vi "Actor Core.vi"(8 "error in":errorcluster, 11 "Example View in":refnum<class "Example View Actor 2.lvclass">) -> (0 "error out":errorcluster, 3 "Actor out":refnum<class "Actor.lvclass">)   [LabVIEW 2023, in "Example Event Actors.lvlib" / "Example View Actor 2.lvlib" / "Example View Actor 2.lvclass"]
doc: "(<B>Filename</B>: Actor Framework.lvlib:Actor.lvclass:Actor Core.vi)\n\nReceives messages to the actor, reacts to them, and initiates any error handling that may shut the actor down.\n\nDescendant classes may override this VI to append parallel tasks for the actor to complete while it handles messages. Overrides use the Call Parent Method node."
uses:
  Example View Actor 2.lvclass
  C:/Program Files/National Instruments/LabVIEW 2023/vi.lib/ActorFramework/Actor/Actor.lvclass
  C:/Projects/Shared Libraries/Event Actors/View Actor/View Actor.lvclass
  <vilib>/ActorFramework/Actor/Actor.lvclass
  Example View Actor 2.lvclass/Example View Actor 2.ctl
  <vilib>/ActorFramework/Actor/Actor.lvclass/Actor.ctl
  <vilib>/ActorFramework/Message Enqueuer/Message Enqueuer.lvclass/Message Enqueuer.ctl
  View Actor/View Actor.lvclass/View Actor.ctl
  Example Events/Boolean Event.lvclass
  C:/Projects/Shared Libraries/Event Actors/Event Data Types/Event Boolean/Event Boolean.lvclass
  C:/Projects/Shared Libraries/Event Actors/Event/Event.lvclass
  View Actor/properties/Read Name.vi
  <vilib>/ActorFramework/Message Enqueuer/Init from Existing Queue.vi
  <vilib>/ActorFramework/Message Enqueuer/Message Enqueuer.lvclass
  View Actor/View Actor.lvclass
  View Actor Messages/Generate and Broadcast Event Msg/Generate and Broadcast Event Msg.lvclass
  C:/Projects/Shared Libraries/Event Actors/Examples/Example View Actor/Example View Actor 2/Example View Actor 2.lvclass
  C:/Projects/Shared Libraries/Event Actors/Examples/Example Events/Boolean Event.lvclass
panel:
  out "View Name":string
  in  "Boolean":bool
  # "This View is not automatically launched by the Controller but  launched manually from the Controller GUI. This View registers only to the Boolean event by calling the Controller's method \"Register by Name.vi\" with the option \"Get Last Broadcast Event (F)\"  set to true. This means that, if the Boolean event was previously fired either by the Controller or by one of the Views, when this View inits the Controller will generate the latest broadcast value of such event to this View. \n\nInstrunctions:\n1. Launch the example\n2. From one of the Views set the Boolean controller to true\n3. From the Controller launch this view\n4. Observe in this VIew that the Boolean control is set to true\n5. Repeat the same forcedure omitting step 2. and observe that the Boolean controller  is set to false"
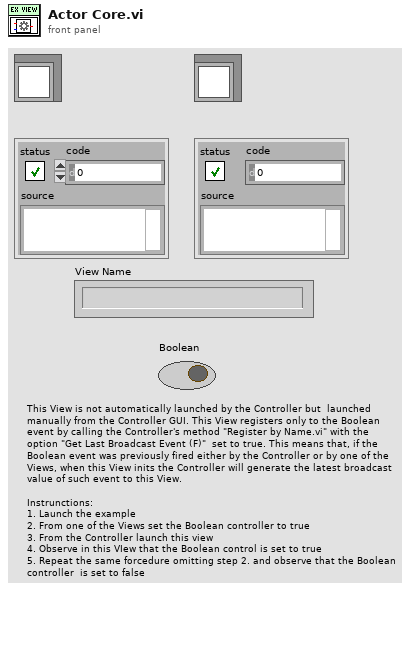
[diagram p1: front panel]
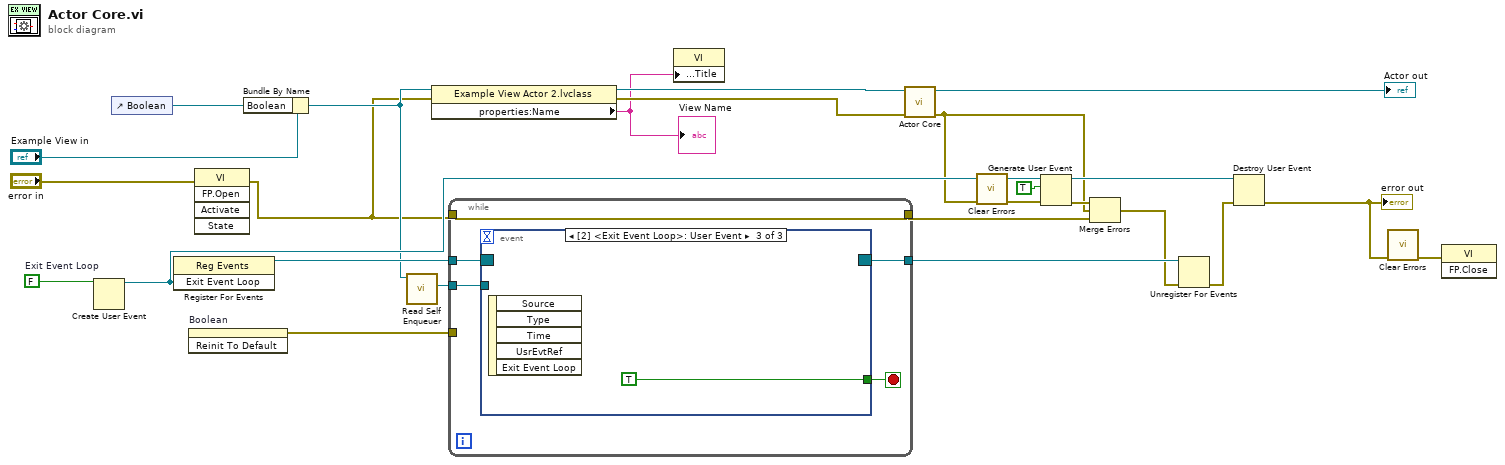
[diagram p0: block diagram]
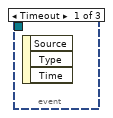
[diagram p2: hidden frame]
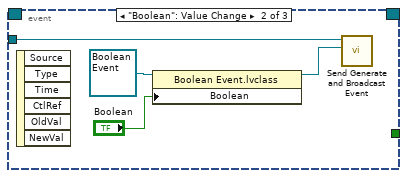
[diagram p3: hidden frame]
diagram:
  w20 = FALSE  # Exit Event Loop
  n1 = Create User Event(user event datatype=w20) -> (user event=w17:refnum<user-event>)  [unwired: 1 in, 1 out]
  n2 = control-ref of="Boolean"() -> (w23:refnum<vi>)
  n3 = register-events(w17) -> (reference out=w19:refnum<event-registration>)  [unwired: 2 in, 1 out]
  n4 = invoke on="Boolean" class="Bool (strict)" method="Reinit To Default"() -> (error out=w1:errorcluster)  [unwired: 3 in, 2 out]
  n5 = invoke class="VI" method="FP.Open"(error in="error in") -> (error out=w4:errorcluster)  [unwired: 4 in, 4 out]
  n6 = Bundle By Name(cluster="Example View in", "Boolean"=w23) -> (w12:refnum<class "Example View Actor 2.lvclass">)
  n7 = call <vilib>:"Read Self Enqueuer.vi"("Actor"=w12) -> ("Self Enqueuer"=w21:refnum<class "Message Enqueuer.lvclass">)  [unwired: 10 in]
  n8 = property class="Example View Actor 2.lvclass"(reference=w12, error in=w4) -> (reference out=w5:refnum<class "Example View Actor 2.lvclass">, error out=w3:errorcluster, "properties:Name"=w2:string)
  "View Name" <- w2
  n9 = while {
    tunnel: w21 -> [w30]
    tunnel: w19 -> [w29]
    tunnel: w4 -> [w28]
    tunnel: [w28] -> w11
    tunnel: [w27] -> w15
    tunnel: w1 -> [_]
    stop <- w26 stop-if-true
    n10 = event shown="[2] <Exit Event Loop>: User Event" {
      selector: w29 -> [_ _ _]
      dyn-events: [_ _ _] -> w27
      timeout: _ -> [_ _ _]
      tunnel: w30 -> [_ w34 _]
      tunnel: [_ _ TRUE] -> w26
      event Timeout {
        n11 = event-data() -> ()  [unwired: 1 in, 3 out]
      }
      event "Boolean": Value Change {
        n12 = event-data() -> ()  [unwired: 1 in, 6 out]
        n13 = property class="Boolean Event.lvclass"(reference=refnum<class "Boolean Event.lvclass"> refnum ("Example Source.lvlib:Boolean Event.lvclass"), "Boolean"="Boolean") -> (reference out=w31:refnum<class "Boolean Event.lvclass">)  [unwired: 1 in, 1 out]
        n14 = call "Send Generate and Broadcast Event.vi"("Event Data"=w31, "Message Enqueuer in"=w34) -> ()  [unwired: 8 in, 2 out]
      }
      event User Event {
        n15 = event-data() -> ()  [unwired: 1 in, 5 out]
      }
    }
  }
  n16 = property class="VI"("Front Panel.Title"=w2) -> ()  [unwired: 2 in, 2 out]
  n17 = call-parent "Actor Core.vi"("error in"=w3, "Actor in"=w5) -> ("error out"=w7:errorcluster, "Actor out"=→"Actor out":refnum<class "Actor.lvclass">)  [unwired: 8 in]
  n18 = call <vilib>:"Clear Errors.vi"("error in (no error)"=w7) -> ("error out"=w6:errorcluster)  [unwired: 5 in, 1 out]
  n19 = Generate User Event(user event=w17, event data cluster=TRUE ("event data"), error in=w6) -> (user event out=w16:refnum<user-event>, error out=w18:errorcluster)  [unwired: 1 in]
  n20 = Merge Errors(w18, w7, w11) -> (w8:errorcluster)
  n21 = Unregister For Events(event registration refnum=w15, error in=w8) -> (error out=w14:errorcluster)
  n22 = Destroy User Event(user event=w16, error in=w14) -> (error out=w9:errorcluster)
  "error out" <- w9
  n23 = call <vilib>:"Clear Errors.vi"("error in (no error)"=w9) -> ("error out"=w10:errorcluster)  [unwired: 5 in, 1 out]
  n24 = invoke class="VI" method="FP.Close"(error in=w10) -> ()  [unwired: 2 in, 3 out]
